vi "AcquisitionLoop.vi"(8 "error in (no error)":errorcluster, 10 "ManualModeQueue":refnum<queue>, 11 "AcquisitionQueue":refnum<queue>) -> (0 "Error Out":errorcluster)   [LabVIEW 2019, in "ManualMode.lvlib"]
uses:
  ManualMode.lvlib
  Cluster - ManualModeMonitorMessage.ctl
  Enum - ManualModeMonitorState.ctl
  Cluster - ManualModeMessageCluster.ctl
  Enum - ManualModeMessage.ctl
  Cluster - UIRefs.ctl
  Mark10 API/ReadTravelAndForce.vi
  Mark10 API/Mark 10 TSTM-DC.lvlib
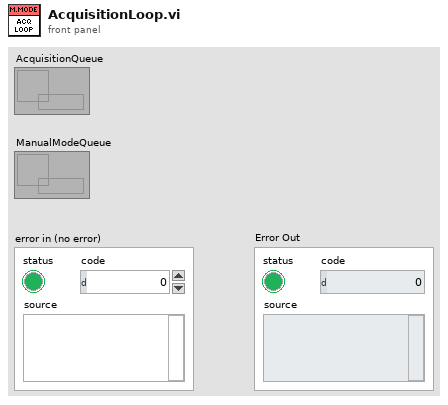
[diagram p1: front panel]
types:
  T1 = typedef "ManualMode.lvlib/Cluster - UIRefs.ctl" = cluster{"Work":refnum<vi>, "Torque":refnum<vi>, "Position":refnum<vi>, "Wf":refnum<vi>}
  T2 = typedef "ManualMode.lvlib/Enum - ManualModeMonitorState.ctl" = enum16{"Idle", "SetCOM", "SetUIRefs", "Start", "Read", "Stop", "Pause", "Exit"}
  T3 = typedef "ManualMode.lvlib/Cluster - ManualModeMonitorMessage.ctl" = cluster{"Message":T2, "Data":variant}
  T4 = typedef "ManualMode.lvlib/Enum - ManualModeMessage.ctl" = enum16{"Initialize", "Idle", "Start", "Stop", "Pause", "Resume", "BroadcastPreCollection", "MoveCCW", "MoveCW", "StopMove", "SetZero", "GotoZero", "UpdateHW", "Error", "Exit"}
  T5 = typedef "Mark 10 TSTM-DC.lvlib/Cluster - FeedbackData.ctl" = cluster{"Angle":dbl, "Torque":dbl, "Work":dbl}
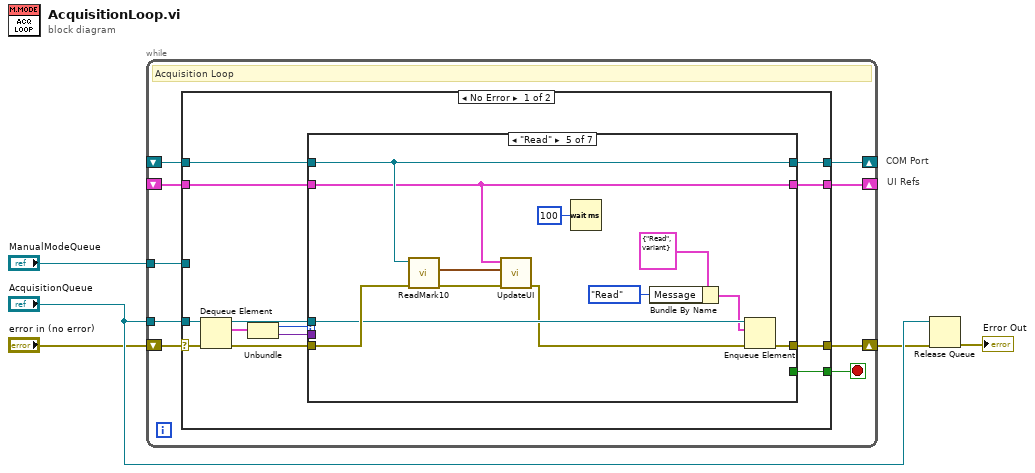
[diagram p0: block diagram]
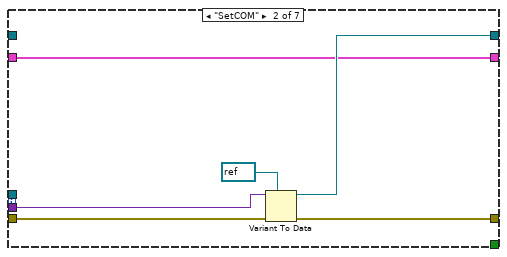
[diagram p3: hidden frame]
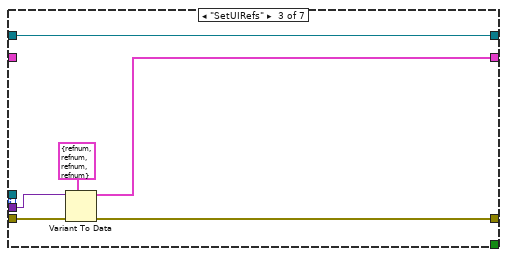
[diagram p4: hidden frame]
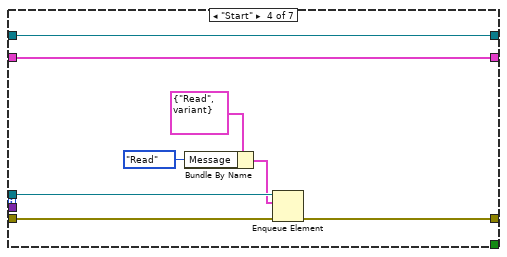
[diagram p5: hidden frame]
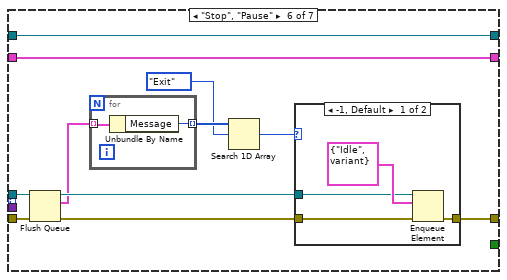
[diagram p6: hidden frame]
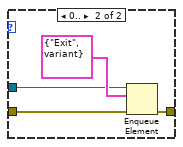
[diagram p7: hidden frame]
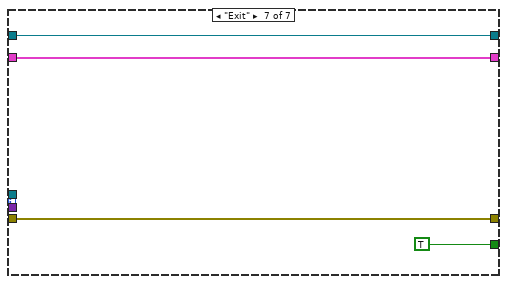
[diagram p8: hidden frame]
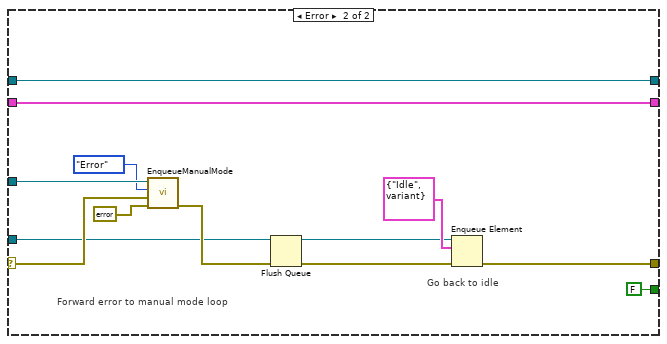
[diagram p9: hidden frame]
diagram:
  # "UI Refs"
  # "COM Port"
  n1 = while {
    tunnel: "AcquisitionQueue" -> [w13]
    shift-right: [w12] -> _
    shift-left: _ -> [w11]
    shift-right: [w9] -> w4
    shift-left: "error in (no error)" -> [w14]
    tunnel: "ManualModeQueue" -> [w8]
    shift-right: [w7] -> _
    shift-left: _ -> [w6]
    stop <- w10 stop-if-true
    # "Acquisition Loop"
    n2 = case shown="No Error" w14 {
      selector: w14 -> [w27 w98]
      tunnel: w13 -> [w26 w90]
      tunnel: [w22 w96] -> w12
      tunnel: w11 -> [w21 w96]
      tunnel: [w20 FALSE] -> w10
      tunnel: [w19 w94] -> w9
      tunnel: w8 -> [_ w99]
      tunnel: [w17 w92] -> w7
      tunnel: w6 -> [w16 w92]
      frame No Error {
        n3 = Dequeue Element(queue=w26, error in (no error)=w27) -> (queue out=w18:refnum<queue>, element=w25:T3, error out=w23:errorcluster)  [unwired: 1 in, 1 out]
        n4 = Unbundle(w25) -> ("Message"=w15:T2, "Data"=w24:variant)
        n5 = case shown="\"Read\"" w15 {
          tunnel: w24 -> [_ w35 w39 _ _ _ _]
          tunnel: w23 -> [w29 w36 w41 w49 w62 w72 w85]
          tunnel: [w30 w34 w42 w50 w61 w73 w87] -> w22
          tunnel: w21 -> [w30 _ w42 w50 w61 w73 w87]
          tunnel: [_ _ _ _ _ _ TRUE] -> w20
          tunnel: [w29 w32 w40 w48 w59 w71 w85] -> w19
          tunnel: w18 -> [_ _ _ w47 w58 w68 _]
          tunnel: [w28 w31 w37 w46 w57 w70 w84] -> w17
          tunnel: w16 -> [w28 w31 _ w46 w57 w70 w84]
          frame "Idle", Default {
          }
          frame "SetCOM" {
            n6 = Variant To Data(error in=w36, type=refnum<visa-resource-name> refnum ("Hardware Configuration.Mark10COM"), Variant=w35) -> (data=w34:refnum<visa-resource-name>, error out=w32:errorcluster)
          }
          frame "SetUIRefs" {
            n7 = Variant To Data(error in=w41, type=T1 {"Work"=refnum, "Torque"=refnum, "Position"=refnum, "Wf"=refnum} ("ManualModeUIRefs"), Variant=w39) -> (data=w37:T1, error out=w40:errorcluster)
          }
          frame "Start" {
            n8 = Bundle By Name(cluster=T3 {"Message"=enum."Read", "Data"=variant} ("element"), "Message"=Enum_-_ManualModeMonitorState."Read") -> (w44:T3)
            n9 = Enqueue Element(queue=w47, element=w44, error in (no error)=w49) -> (error out=w48:errorcluster)  [unwired: 1 in, 2 out]
          }
          frame "Read" {
            n10 = call-poly "ReadMark10.vi"("error in"=w62, "VISA resource name"=w61) -> ("error out"=w55:errorcluster, "FeedbackData"=w56:T5)  [unwired: 7 in, 1 out]
            n11 = call "UpdateUI.vi"("Error In"=w55, "FeedbackData"=w56, "ManualModeUIRefs"=w57) -> ("Error Out"=w54:errorcluster)  [unwired: 8 in]
            n12 = Wait (ms)(milliseconds to wait=u32 100) -> ()  [unwired: 1 out]
            n13 = Bundle By Name(cluster=T3 {"Message"=enum."Read", "Data"=variant} ("element"), "Message"=Enum_-_ManualModeMonitorState."Read") -> (w51:T3)
            n14 = Enqueue Element(queue=w58, element=w51, error in (no error)=w54) -> (error out=w59:errorcluster)  [unwired: 1 in, 2 out]
          }
          frame "Stop", "Pause" {
            n15 = Flush Queue(queue=w68, error in (no error)=w72) -> (queue out=w67:refnum<queue>, remaining elements=w66:T3[], error out=w69:errorcluster)
            n16 = for {
              tunnel: w66 -> [w83] mode=indexing
              tunnel: [w82] -> w65 mode=indexing
              n17 = Unbundle By Name(w83) -> ("Message"=w82:T2)
            }
            n18 = Search 1D Array(1D array=w65, element=Enum_-_ManualModeMonitorState."Exit") -> (index of element=w63:i32)  [unwired: 1 in]
            n19 = case shown="-1, Default" w63 {
              tunnel: [w77 w81] -> w71
              tunnel: w69 -> [w75 w79]
              tunnel: w67 -> [w74 w78]
              frame -1, Default {
                n20 = Enqueue Element(queue=w74, element=T3 {"Message"=enum."Idle", "Data"=variant}, error in (no error)=w75) -> (error out=w77:errorcluster)  [unwired: 1 in, 2 out]
              }
              frame 0.. {
                n21 = Enqueue Element(queue=w78, element=T3 {"Message"=enum."Exit", "Data"=variant}, error in (no error)=w79) -> (error out=w81:errorcluster)  [unwired: 1 in, 2 out]
              }
            }
          }
          frame "Exit" {
          }
        }
      }
      frame Error {
        # "Go back to idle"
        # "Forward error to manual mode loop"
        n22 = call "EnqueueManualMode.vi"("error in (no error)"=errorcluster {"status"=FALSE, "code"=0, "source"=""}, "Data"=w98, "Message"=Enum_-_ManualModeMessage."Error", "queue"=w99) -> ("error out"=w100:errorcluster)  [unwired: 6 in, 1 out]
        n23 = Flush Queue(queue=w90, error in (no error)=w100) -> (queue out=w89:refnum<queue>, error out=w91:errorcluster)  [unwired: 1 out]
        n24 = Enqueue Element(queue=w89, element=T3 {"Message"=enum."Idle", "Data"=variant}, error in (no error)=w91) -> (error out=w94:errorcluster)  [unwired: 1 in, 2 out]
      }
    }
  }
  n25 = Release Queue(queue="AcquisitionQueue", error in (no error)=w4) -> (error out=→"Error Out":errorcluster)  [unwired: 1 in, 2 out]
